vi "Initialize.vi"(8 "error in":errorcluster, 10 "shared resources":refnum<class "Shared Resources.lvclass">, 11 "Tx UDP Execution Unit in":refnum<class "Tx UDP Execution Unit.lvclass">) -> (0 "error out":errorcluster, 3 "Tx UDP Execution Unit out":refnum<class "Tx UDP Execution Unit.lvclass">)   [LabVIEW 2020, in "AIM ARINC 664 Engine.lvlib" / "Implementation.lvlib" / "Tx UDP Execution Unit.lvclass"]
uses:
  Tx UDP Execution Unit.lvclass
  Tx UDP Execution Unit.lvclass/Tx UDP Execution Unit.ctl
  <instrlib>/AIM GmbH/_AIM 664/AIM664LV.lvlib
  <instrlib>/AIM GmbH/_AIM 664/bsp/Fdx Create Session (Tx-UDP Port-Oriented).vi
  <instrlib>/AIM GmbH/_AIM 664/bsp/Transmit/FdxCreateTxVL.vi
  <instrlib>/AIM GmbH/_AIM 664/bsp/Fdx Create UDP Port (TX-CommPort).vi
  <vilib>/Utility/SystemLogging/NI_SystemLogging.lvlib
  Interfaces/Shared Resources/Shared Resources.lvclass
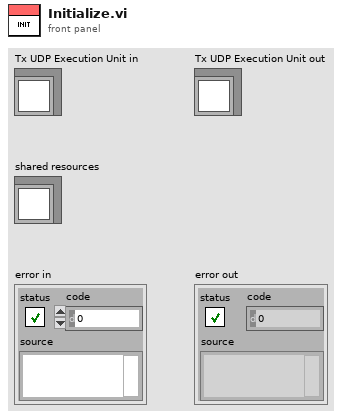
[diagram p1: front panel]
types:
  T1 = typedef "AIM664LV.lvlib/comm_config_vl_tx.ctl" = cluster{"VlId":u16, "NumOfSubVl":u16, "rate ms [Bag]":u32, "domainID":u8, "sideID":u8, "locationID":u8, "interfaceID":u8, "NetSelect":u32, "Skew":u32, "MaxFrameLength":u32, "FrameBufferSize":u32}
  T2 = typedef "AIM664LV.lvlib/comm_udp_tx.ctl" = cluster{"PortType":enum16{"FDX_UDP_SAMPLING", "FDX_UDP_QUEUING"}, "partitionID":u8, "SubVlId":u8, "UdpSrcPort":u16, "UdpDstPort":u16, "SampleRateMs":dbl, "UdpNumBufMessages":u32, "UdpMaxMessageSize":u32}
  T3 = cluster{"VL Config":T1, "CommPort Config":T2[]}[]
  T4 = typedef "EthFrameManagement.lvlib/arinc664_mac_src_info.ctl" = cluster{"domainID":u8, "sideID":u8, "locationID":u8, "interfaceID":u8}
  T5 = typedef "Encoding (Arinc664).ctl" = u16
  T6 = cluster{"Data":u8[], "Parameters":cluster{"start index":i32, "size":i32, "encoding":T5, "signed":bool, "scale multiplier":dbl, "scale offset":dbl}[]}[]
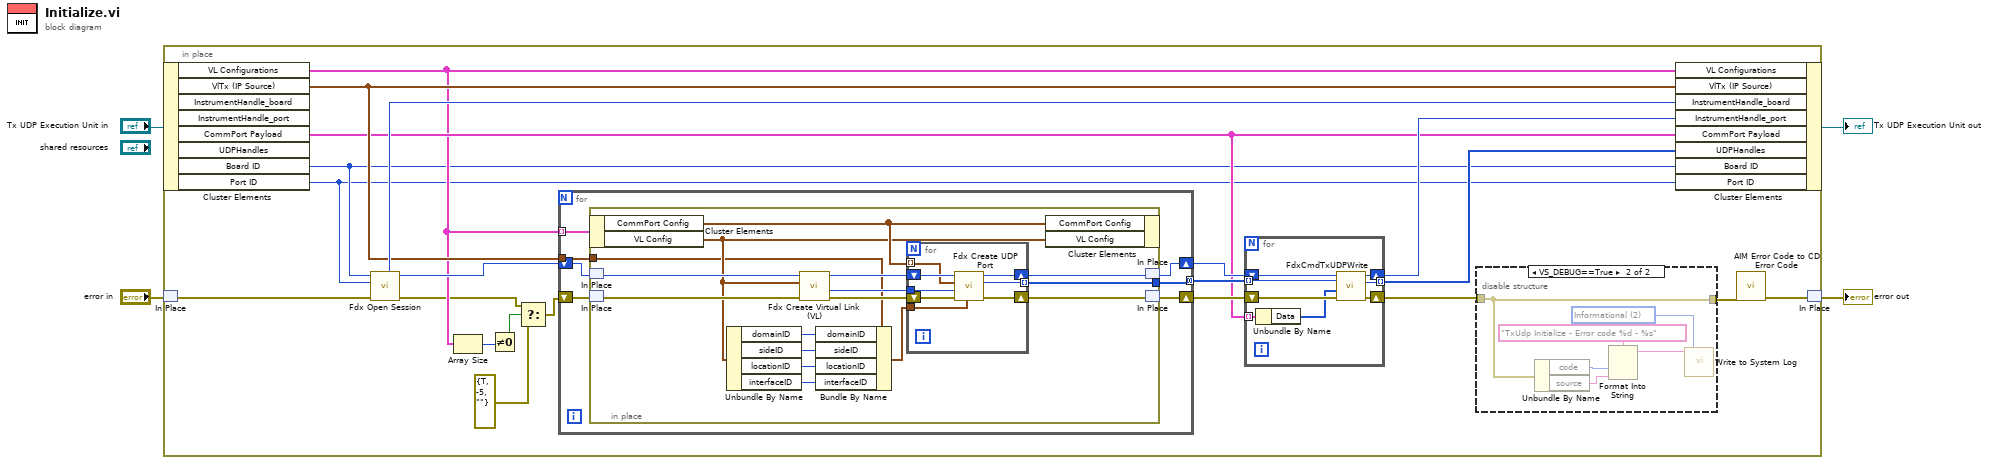
[diagram p0: block diagram]
diagram:
  n1 = in-place {
    n2 = in-place-cluster #1("Tx UDP Execution Unit in") -> ("VL Configurations"=w15:T3, "VlTx (IP Source)"=w19:T4, "CommPort Payload"=w16:T6, "Board ID"=w9:u32, "Port ID"=w8:u32)  [unwired: 3 out]
    n3 = in-place-match #2("error in") -> (w25:errorcluster)
    n4 = call-poly <instrlib>:"Fdx Open Session.vi"("error in (no error)"=w25, "port"=w8, "board"=w9) -> ("error out"=w12:errorcluster, "port handle out"=w22:u32, "InstrumentHandle_board out"=w23:u32)  [unwired: 4 in, 2 out]
    n5 = Array Size(array=w15) -> (size(s)=w14:i32)
    n6 = Not Equal To 0?(x=w14) -> (x != 0?=w13:bool)
    n7 = Select(t=w12, s=w13, f=errorcluster {"status"=TRUE, "code"=-5, "source"=""}) -> (s? t:f=w11:errorcluster)
    n8 = for {
      tunnel: w15 -> [w31] mode=indexing
      shift-right: [w29] -> w21
      shift-left: w22 -> [w30]
      shift-right: [w28] -> w24
      shift-left: w11 -> [w32]
      tunnel: w19 -> [w27]
      tunnel: [w26] -> w18 mode=concatenating
      n9 = in-place {
        in-place-border: w27 -> [w38]
        in-place-border: [w41] -> w26
        n10 = in-place-cluster #3(w31) -> ("CommPort Config"=w44:T2[], "VL Config"=w39:T1)
        n11 = in-place-match #4(w30) -> (w47:u32)
        n12 = in-place-match #5(w32) -> (w48:errorcluster)
        n13 = Unbundle By Name(w39) -> ("domainID"=w37:u8, "sideID"=w36:u8, "locationID"=w35:u8, "interfaceID"=w34:u8)
        n14 = call-poly <instrlib>:"Fdx Create Virtual Link (VL).vi"("error in (no error)"=w48, "VL Config"=w39, "InstrumentHandle in"=w47) -> ("error out"=w46:errorcluster, "VlId"=w40:u16, "InstrumentHandle out"=w45:u32)  [unwired: 6 in]
        n15 = Bundle By Name(cluster=w38, "domainID"=w37, "sideID"=w36, "locationID"=w35, "interfaceID"=w34) -> (w33:T4)
        n16 = for {
          shift-right: [w49] -> w43
          shift-left: w46 -> [w56]
          shift-right: [w51] -> w42
          shift-left: w45 -> [w55]
          tunnel: w44 -> [w54] mode=indexing
          tunnel: [w50] -> w41 mode=indexing
          tunnel: w33 -> [w53]
          tunnel: w40 -> [w52]
          n17 = call-poly <instrlib>:"Fdx Create UDP Port.vi"("VlTx"=w53, "error in"=w56, "VlId"=w52, "CommPort Config"=w54, "port handle in"=w55) -> ("error out"=w49:errorcluster, "commPort handle out"=w50:u32, "port handle out"=w51:u32)  [unwired: 3 in, 1 out]
        }
        n18 = in-place-cluster #3("CommPort Config"=w44, "VL Config"=w39) -> ()  [unwired: 1 out]
        n19 = in-place-match #4(w42) -> (w29:u32)
        n20 = in-place-match #5(w43) -> (w28:errorcluster)
      }
    }
    n21 = for {
      shift-right: [w63] -> w6
      shift-left: w24 -> [w64]
      shift-right: [w61] -> w20
      shift-left: w21 -> [w62]
      tunnel: w18 -> [w60] mode=indexing
      tunnel: [w59] -> w17 mode=indexing
      tunnel: w16 -> [w58] mode=indexing
      n22 = Unbundle By Name(w58) -> ("Data"=w57:u8[])
      n23 = call <instrlib>:"FdxCmdTxUDPWrite.vi"("error in"=w64, "Data"=w57, "UdpHandle"=w60, "InstrumentHandle"=w62) -> ("error out"=w63:errorcluster, "UdpHandleOut"=w59:u32, "InstrumentHandle"=w61:u32)  [unwired: 4 in, 1 out]
    }
    n24 = disable-structure shown="VS_DEBUG==True" {
      disable-tunnel: w6 -> [w65 w66]
      disable-tunnel: [w65 w66] -> w5
      frame condition #0 (active) {
      }
      frame condition #1 {
        w69 = 2 items=["Error", "Warning", "Informational"] ("severity")
        n25 = Unbundle By Name(w66) -> ("code"=w68:i32, "source"=w67:string)
        n26 = Format Into String(format string="TxUdp Initialize - Error code %d - %s", w68, w67) -> (resulting string=w70:string)  [unwired: 2 in, 1 out]
        n27 = call <vilib>:"Write to System Log.vi"("severity"=w69, "message"=w70) -> ()  [unwired: 9 in, 1 out]
      }
    }
    n28 = in-place-cluster #1("VL Configurations"=w15, "VlTx (IP Source)"=w19, "InstrumentHandle_board"=w23, "InstrumentHandle_port"=w20, "CommPort Payload"=w16, "UDPHandles"=w17, "Board ID"=w9, "Port ID"=w8) -> (→"Tx UDP Execution Unit out":refnum<class "Tx UDP Execution Unit.lvclass">)
    n29 = call "AIM Error Code to CD Error Code.vi"("error in"=w5) -> ("error out"=w7:errorcluster)  [unwired: 7 in, 3 out]
    n30 = in-place-match #2(w7) -> (→"error out":errorcluster)
  }
